vi "TreeNode Get TimeInserted.vi"(8 "error in (no error)":errorcluster, 11 "TreeNode DVR in":refnum<data-value>) -> (0 "error out":errorcluster, 1 "TimeInserted String out":string, 2 "timeInsertedOut":i64, 3 "TreeNode DVR out":refnum<data-value>)   [LabVIEW 2015, in "MDSplus.lvlib"]
uses:
  <vilib>/MDSplus/Library/MDSplus.lvlib
  <vilib>/MDSplus/Classes/Data_Class/TreeNode_Class/TreeNode.lvclass
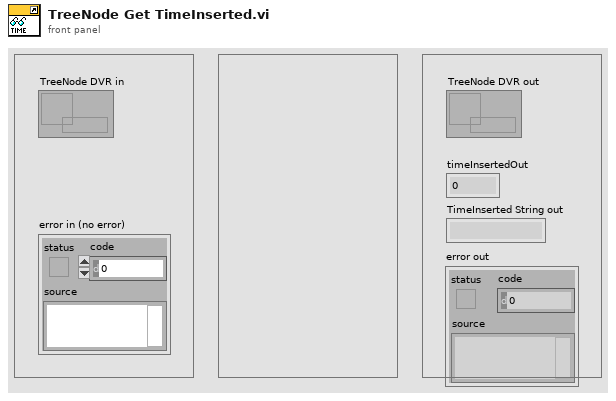
[diagram p1: front panel]
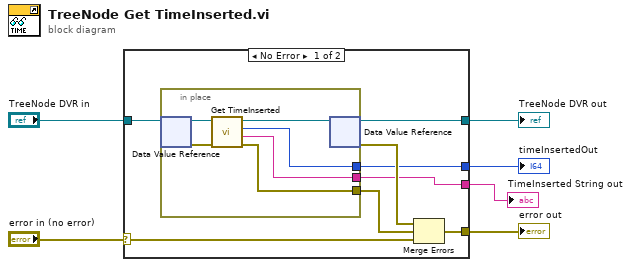
[diagram p0: block diagram]
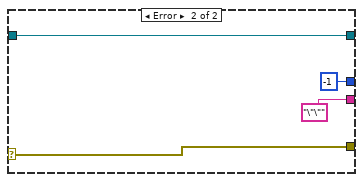
[diagram p2: hidden frame]
diagram:
  n1 = case shown="No Error" "error in (no error)" {
    selector: "error in (no error)" -> [w13 w24]
    tunnel: "TreeNode DVR in" -> [w14 w23]
    tunnel: [w10 w24] -> w6
    tunnel: [w11 w23] -> w3
    tunnel: [w8 i64 -1 ("timeInsertedOut")] -> w2
    tunnel: [w7 "\"\"" ("String value out 2")] -> w1
    frame No Error {
      n2 = in-place {
        in-place-border: [w18] -> w9
        in-place-border: [w16] -> w8
        in-place-border: [w15] -> w7
        n3 = in-place-dvr #1(w14) -> (w20:refnum<class "TreeNode.lvclass">, w19:errorcluster)
        n4 = call-dynamic "Get TimeInserted.vi"("error in (no error)"=w19, "TreeNode in"=w20) -> ("error out"=w18:errorcluster, "TimeInserted String out"=w15:string, "timeInsertedOut"=w16:i64, "TreeNode out"=w17:refnum<class "TreeNode.lvclass">)  [unwired: 6 in]
        n5 = in-place-dvr #1(w17) -> (w11:refnum<data-value>, w12:errorcluster)
      }
      n6 = Merge Errors(w12, w9, w13) -> (w10:errorcluster)
    }
    frame Error {
    }
  }
  "error out" <- w6
  "TreeNode DVR out" <- w3
  "timeInsertedOut" <- w2
  "TimeInserted String out" <- w1
